vi "Status.get.vi"(8 "error in (no error)":errorcluster, 11 "comic_crawler in":refnum<class "comic_crawler.lvclass">) -> (0 "error out":errorcluster, 2 "current status":T1, 3 "comic_crawler out":refnum<class "comic_crawler.lvclass">)   [LabVIEW 2024, in "comic_crawler.lvclass"]
uses:
  comic_crawler.lvclass
  comic_crawler.lvclass/comic_crawler.ctl
  status--cluster.ctl
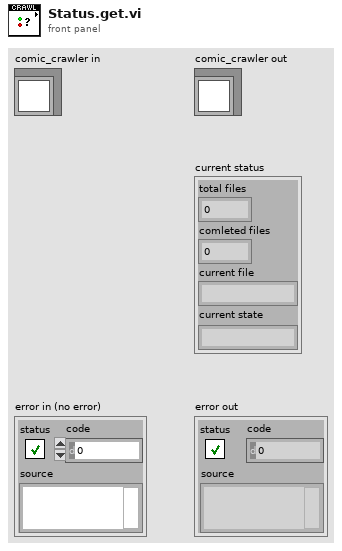
[diagram p1: front panel]
types:
  T1 = typedef "comic_crawler.lvclass/status--cluster.ctl" = cluster{"total files":i32, "comleted files":i32, "current file":string, "current state":string}
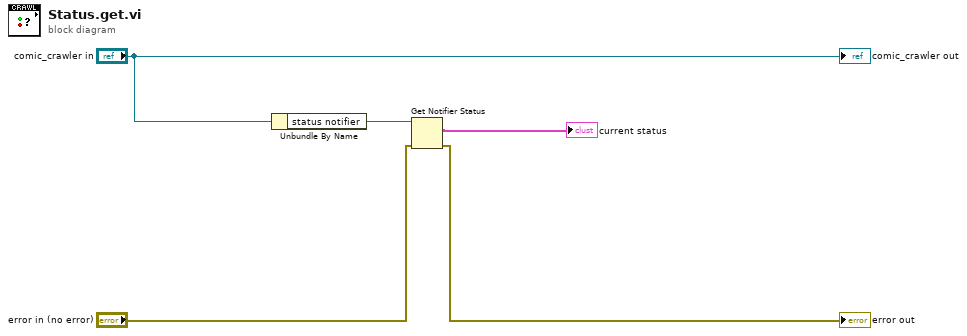
[diagram p0: block diagram]
diagram:
  n1 = Unbundle By Name("comic_crawler in") -> ("status notifier"=w4:refnum<notifier>)
  n2 = Get Notifier Status(notifier=w4, error in (no error)="error in (no error)") -> (current notification=→"current status":T1, error out=→"error out":errorcluster)  [unwired: 3 out]
  "comic_crawler out" <- "comic_crawler in"
